vi "Integral.vi"(1 "En rango?":bool, 2 "KI":dbl, 3 "Dt":dbl, 4 "Error":dbl) -> (0 "Acción Integral":dbl)   [LabVIEW 2011]
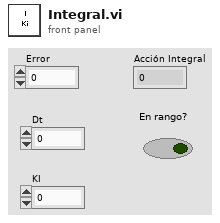
[diagram p1: front panel]
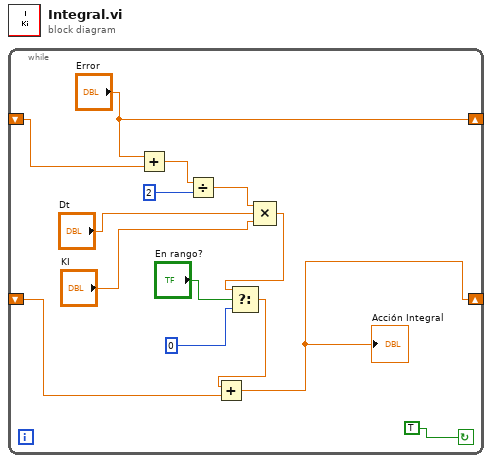
[diagram p0: block diagram]
diagram:
  n1 = while {
    shift-right: ["Error"] -> _
    shift-left: _ -> [w14]
    shift-right: [w11] -> _
    shift-left: _ -> [w10]
    stop <- TRUE continue-if-true
    n2 = Add(x="Error", y=w14) -> (x+y=w12:dbl)
    n3 = Divide(x=w12, y=2) -> (x/y=w8:dbl)
    n4 = Compound Arithmetic op=MULTIPLY(w8, "Dt", "KI") -> (w4:dbl)
    n5 = Select(t=w4, s="En rango?", f=0) -> (s? t:f=w3:dbl)
    n6 = Add(x=w3, y=w10) -> (x+y=w11:dbl)
    "Acción Integral" <- w11
  }
